vi "Configure Transform.vi"(6 "Enable Transform (F: Disable)":bool, 8 "error in (no error)":errorcluster, 9 "Transform Mode (1: Lowpass Step)":i32(ring)=1 items=["Lowpass Impulse", "Lowpass Step", "Bandpass Impulse"], 10 "Channel (1)":i32=1, 11 "VISA resource name":refnum<visa-resource-name>) -> (0 "error out":errorcluster, 3 "VISA resource name out":refnum<visa-resource-name>)   [LabVIEW 2018, in "Keysight PNA Series.lvlib"]
doc: "Configures time domain transform."
uses:
  Keysight PNA Series.lvlib
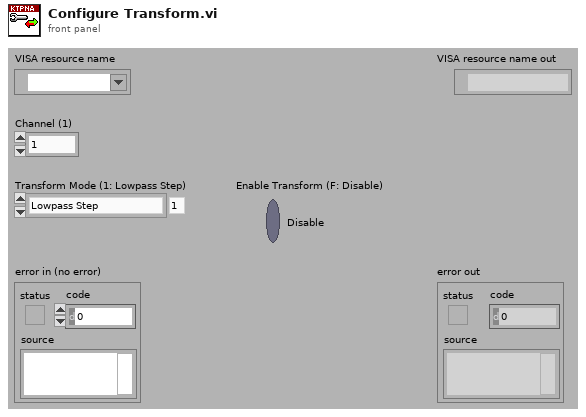
[diagram p1: front panel]
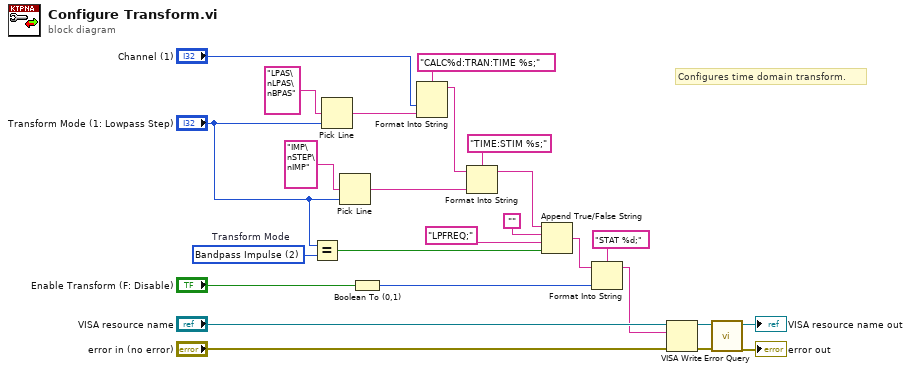
[diagram p0: block diagram]
diagram:
  w5 = 2 items=["Lowpass Impulse", "Lowpass Step", "Bandpass Impulse"]  # Transform Mode
  # "Configures time domain transform."
  n1 = Equal?(x="Transform Mode (1: Lowpass Step)", y=w5) -> (x = y?=w3:bool)
  n2 = Pick Line(multi-line string="LPAS\nLPAS\nBPAS", line index="Transform Mode (1: Lowpass Step)") -> (output string=w22:string)  [unwired: 1 in]
  n3 = Pick Line(multi-line string="IMP\nSTEP\nIMP", line index="Transform Mode (1: Lowpass Step)") -> (output string=w18:string)  [unwired: 1 in]
  n4 = Boolean To (0,1)(Boolean="Enable Transform (F: Disable)") -> (0, 1=w7:i16)
  n5 = Format Into String(format string="CALC%d:TRAN:TIME %s;", "Channel (1)", w22) -> (resulting string=w20:string)  [unwired: 2 in, 1 out]
  n6 = Format Into String(format string="TIME:STIM %s;", initial string=w20, w18) -> (resulting string=w9:string)  [unwired: 1 in, 1 out]
  n7 = Append True/False String(1:w3, 2:"LPFREQ;", 3:"", 4:w9) -> (0:w17:string)
  n8 = Format Into String(format string="STAT %d;", initial string=w17, w7) -> (resulting string=w6:string)  [unwired: 1 in, 1 out]
  n9 = VISA Write(VISA resource name="VISA resource name", write buffer=w6, error in (no error)="error in (no error)") -> (VISA resource name out=w13:refnum<visa-resource-name>, error out=w12:errorcluster)  [unwired: 1 out]
  n10 = call "Error Query.vi"("error in (no error)"=w12, "VISA resource name"=w13) -> ("error out"=→"error out":errorcluster, "VISA resource name out"=→"VISA resource name out":refnum<visa-resource-name>)  [unwired: 6 in, 2 out]
